vi "Robot Global Data.vi"() -> ()   [LabVIEW 2016]
doc: "This global VI can contain as many global variables as you need. Place a control on the panel, give it a good name. To read or write to it from a VI, drag the icon to the diagram of that VI. You can also drag from the project. Click on the node to change which global you access. You shouldn't have multiple locations writing to a global or it will cause a race-condition."
uses:
  <vilib>/Rock Robotics/WPI/Camera/WPI_CameraImageSize.ctl
  <vilib>/Rock Robotics/WPI/DriverStation/WPI_DriverStationRobotMode2.ctl
panel:
  out "Distance":dbl
  out "Robot Not Moving?":bool
  out "VisionX":dbl
  out "RightStickBumper":bool
  out "LeftStickBumper":bool
  out "ButtonSelect":bool
  out "ButtonStart":bool
  out "BumperLeft":bool
  out "BumperRight":bool
  out "ButtonY":bool
  out "ButtonB":bool
  out "ButtonA":bool
  out "ButtonX":bool
  out "TriggerLeft":bool
  out "TriggerRight":bool
  out "Rear Right Encoder":dbl
  out "Rear Left Encoder":dbl
  out "Front Right Encoder":dbl
  out "Front Left Encoder":dbl
  out "Rotation":dbl
  out "Y":dbl
  out "X":dbl
  in  "Robot Mode":T1
  in  "image size":T2=enum."320x240"
  in  "Enable Vision":bool
  # "1/17/2017 9:30\nVersion 1"
  # "Version 2.0"
  # "2/11/17 2:15"
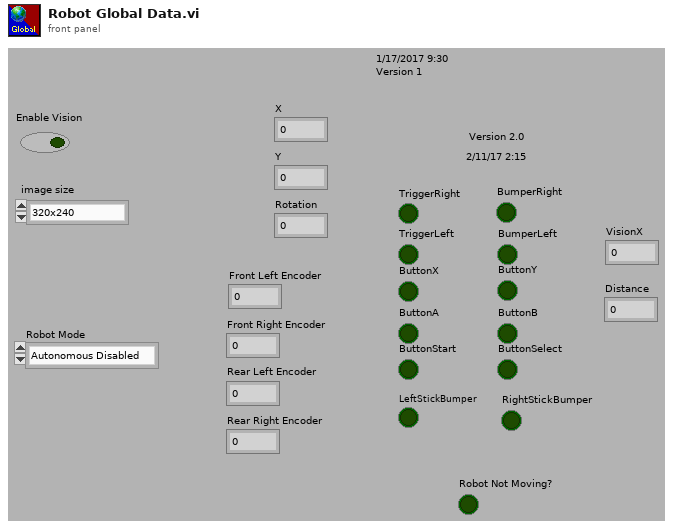
[diagram p1: front panel]
types:
  T1 = typedef "WPI_DriverStationRobotMode2.ctl" = enum16{"Autonomous Disabled", "Autonomous Enabled", "Teleop Disabled", "Teleop Enabled", "Disconnected", "Finish", "Test Disabled", "Test Enabled", "Emergency Stopped"}
  T2 = typedef "WPI_CameraImageSize.ctl" = enum16{"640x480", "320x240", "160x120", "Custom"}
diagram:
